vi "Robocopy_Sub.vi"(5 "Destination Directory":path=path "J:/Paul Hayden/Documents/Personal", 6 "Source Directory":path=path "C:/Users/Paul Hayden/Documents/Personal", 7 "Mode of operation":u16(ring)=2 items=["One way mirror, overwrite destination files even if newer", "One way mirror, don't overwrite newer files at destination", "Two way mirror, newest files at both locations"]) -> ()   [LabVIEW 2014]
panel:
  out "standard output":string
  out "error out":errorcluster
  out "Command String":string
  # "PN 04/11/2014"
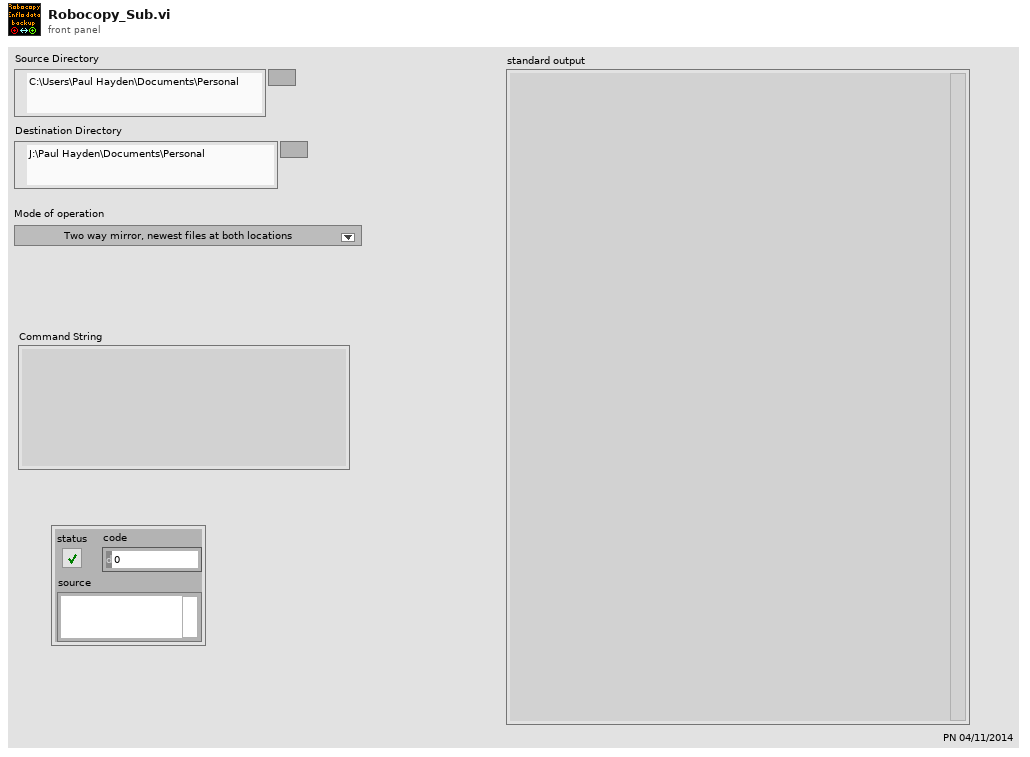
[diagram p1: front panel]
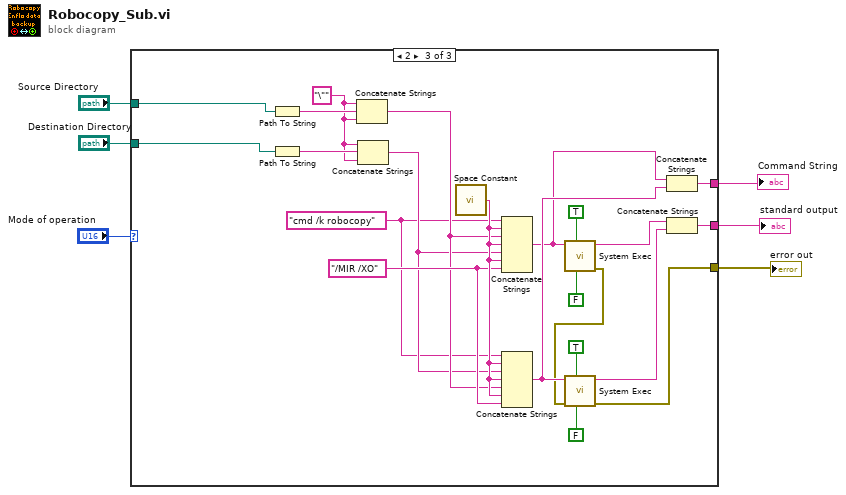
[diagram p0: block diagram]
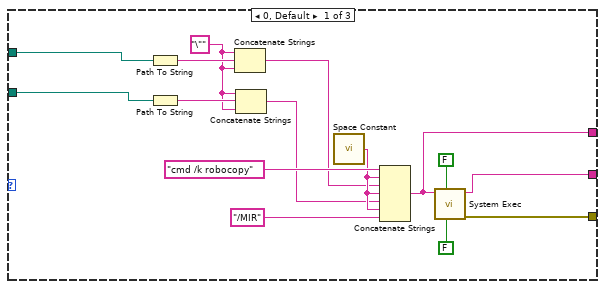
[diagram p2: hidden frame]
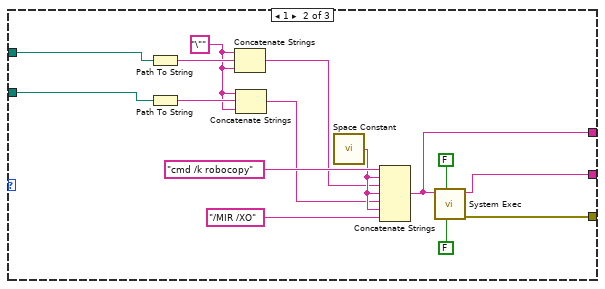
[diagram p3: hidden frame]
diagram:
  n1 = case shown="2" "Mode of operation" {
    tunnel: "Source Directory" -> [w21 w36 w58]
    tunnel: "Destination Directory" -> [w20 w35 w57]
    tunnel: [w19 w34 w50] -> w2
    tunnel: [w18 w33 w56] -> w3
    tunnel: [w17 w32 w53] -> w1
    frame 0, Default {
      w7 = "\"" ("string")
      n2 = Path To String(path=w21) -> (string=w11:string)
      n3 = Path To String(path=w20) -> (string=w9:string)
      n4 = Concatenate Strings(w7, w11, w7) -> (w10:string)
      n5 = Concatenate Strings(w7, w9, w7) -> (w8:string)
      n6 = call <vilib>:"Space Constant.vi"() -> ("String"=w12:string)
      n7 = Concatenate Strings("cmd /k robocopy", w12, w10, w12, w8, w12, "/MIR" ("string")) -> (w19:string)
      n8 = call <vilib>:"System Exec.vi"("run minimized? (F)"=FALSE, "wait until completion? (T)"=FALSE, "command line"=w19) -> ("error out"=w18:errorcluster, "standard output"=w17:string)  [unwired: 5 in, 2 out]
    }
    frame 1 {
      w22 = "\"" ("string")
      n9 = Path To String(path=w36) -> (string=w26:string)
      n10 = Path To String(path=w35) -> (string=w24:string)
      n11 = Concatenate Strings(w22, w26, w22) -> (w25:string)
      n12 = Concatenate Strings(w22, w24, w22) -> (w23:string)
      n13 = call <vilib>:"Space Constant.vi"() -> ("String"=w27:string)
      n14 = Concatenate Strings("cmd /k robocopy", w27, w25, w27, w23, w27, "/MIR /XO" ("string")) -> (w34:string)
      n15 = call <vilib>:"System Exec.vi"("run minimized? (F)"=FALSE, "wait until completion? (T)"=FALSE, "command line"=w34) -> ("error out"=w33:errorcluster, "standard output"=w32:string)  [unwired: 5 in, 2 out]
    }
    frame 2 {
      w45 = "\"" ("string")
      w41 = "/MIR /XO" ("string")
      w38 = "cmd /k robocopy"
      n16 = Path To String(path=w58) -> (string=w47:string)
      n17 = Path To String(path=w57) -> (string=w46:string)
      n18 = Concatenate Strings(w45, w47, w45) -> (w40:string)
      n19 = Concatenate Strings(w45, w46, w45) -> (w39:string)
      n20 = call <vilib>:"Space Constant.vi"() -> ("String"=w42:string)
      n21 = Concatenate Strings(w38, w42, w40, w42, w39, w42, w41) -> (w51:string)
      n22 = Concatenate Strings(w38, w42, w39, w42, w40, w42, w41) -> (w52:string)
      n23 = call <vilib>:"System Exec.vi"("run minimized? (F)"=FALSE, "wait until completion? (T)"=TRUE, "command line"=w51) -> ("error out"=w37:errorcluster, "standard output"=w55:string)  [unwired: 5 in, 2 out]
      n24 = call <vilib>:"System Exec.vi"("run minimized? (F)"=FALSE, "wait until completion? (T)"=TRUE, "error in (no error)"=w37, "command line"=w52) -> ("error out"=w56:errorcluster, "standard output"=w54:string)  [unwired: 4 in, 2 out]
      n25 = Concatenate Strings(w51, w52) -> (w50:string)
      n26 = Concatenate Strings(w55, w54) -> (w53:string)
    }
  }
  "error out" <- w3
  "Command String" <- w2
  "standard output" <- w1
